vi "Index.vi"(8 "error in (no error)":errorcluster, 10 "Index":i32, 11 "Double Array in":refnum<class "Double Array.lvclass">) -> (0 "error out":errorcluster, 3 "Indexed element":refnum<class "Generic Data.lvclass">)   [LabVIEW 2020, in "Data.lvlib" / "Double Array.lvclass"]
doc: "Index an element from 'Generic Data in'.\nThis implementation returns a generic U32 class with the indexed U32."
uses:
  Double Array.lvclass
  Generic Data.lvclass
  Double Array.lvclass/Double Array.ctl
  Double/Double.lvclass/Double.ctl
  Double/Double.lvclass
  C:/Users/Henri/OneDrive/LabVIEW/Framework/Data/Generic Data/Generic Data.lvclass
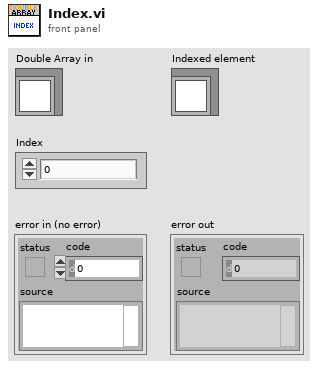
[diagram p1: front panel]
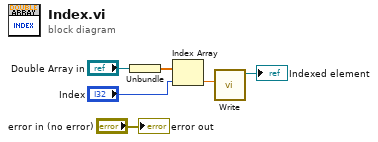
[diagram p0: block diagram]
diagram:
  n1 = Unbundle("Double Array in") -> (w5:dbl[])
  n2 = Index Array(array=w5, index="Index") -> (element=w2:dbl)
  n3 = call "Write.vi"("Double"=w2) -> ("Double out"=→"Indexed element":refnum<class "Double.lvclass">)  [unwired: 10 in]
  "error out" <- "error in (no error)"
